vi "LED.Set.vi"(7 "mode":enum16{"init", "set", "uninit"}(ring)=enum."set", 8 "error in":errorcluster, 10 "LED":bool) -> (0 "error out":errorcluster)   [LabVIEW 2020]
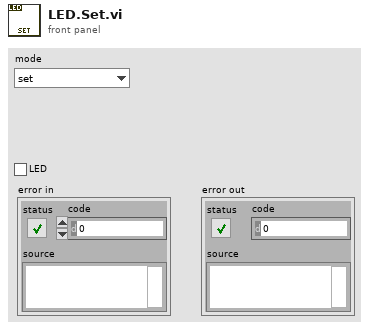
[diagram p1: front panel]
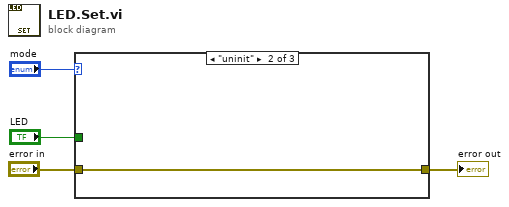
[diagram p0: block diagram]
diagram:
  n1 = case shown="\"uninit\"" "mode" {
    tunnel: "error in" -> [w4 w5 w6]
    tunnel: [w4 w5 w6] -> _
    tunnel: "LED" -> [_ _ _]
    frame "set" {
    }
    frame "uninit" {
    }
    frame "init" {
    }
  }
  "error out" <- "error in"
